vi "Init Sync Box.vi"(8 "error in (no error)":errorcluster, 11 "SPARC4_GUI in":refnum<class "SPARC4_GUI.lvclass">) -> (0 "error out":errorcluster, 3 "SPARC4_GUI out":refnum<class "SPARC4_GUI.lvclass">)   [LabVIEW 2018, in "SPARC4_GUI.lvclass"]
uses:
  SPARC4_GUI.lvclass
  SPARC4_GUI.lvclass/SPARC4_GUI.ctl
  Sync Box/Sync Box.lvclass
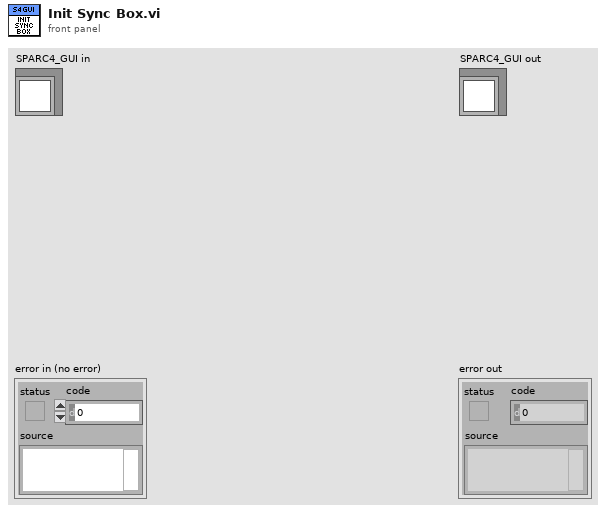
[diagram p1: front panel]
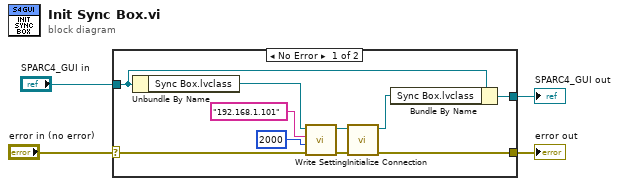
[diagram p0: block diagram]
diagram:
  n1 = case shown="No Error" "error in (no error)" {
    selector: "error in (no error)" -> [w12 w16]
    tunnel: [w10 w16] -> w3
    tunnel: [w13 w15] -> w1
    tunnel: "SPARC4_GUI in" -> [w14 w15]
    frame No Error {
      n2 = Unbundle By Name(w14) -> ("Sync Box.lvclass"=w7:refnum<class "Sync Box.lvclass">)
      n3 = call "Write Setting.vi"("error in (no error)"=w12, "Remote Port"=u32 2000, "Address"="192.168.1.101", "Sync Box in"=w7) -> ("error out"=w11:errorcluster, "Sync Box out"=w8:refnum<class "Sync Box.lvclass">)  [unwired: 6 in]
      n4 = call "Initialize Connection.vi"("error in (no error)"=w11, "Sync Box in"=w8) -> ("error out"=w10:errorcluster, "Sync Box out"=w9:refnum<class "Sync Box.lvclass">)  [unwired: 7 in, 1 out]
      n5 = Bundle By Name(cluster=w14, "Sync Box.lvclass"=w9) -> (w13:refnum<class "SPARC4_GUI.lvclass">)
    }
    frame Error {
    }
  }
  "error out" <- w3
  "SPARC4_GUI out" <- w1
